vi "Get-velocity-profile.vi"(8 "error in (no error)":errorcluster, 11 "Motor-Maxon in":refnum<class "Motor-Maxon.lvclass">) -> (0 "error out":errorcluster, 1 "Velocity":i32, 2 "Velocity profile":T1, 3 "Motor-Maxon out":refnum<class "Motor-Maxon.lvclass">)   [LabVIEW 2013, in "PowderDeposition.lvlib" / "Motor-Maxon.lvclass"]
uses:
  Motor-Maxon.lvclass
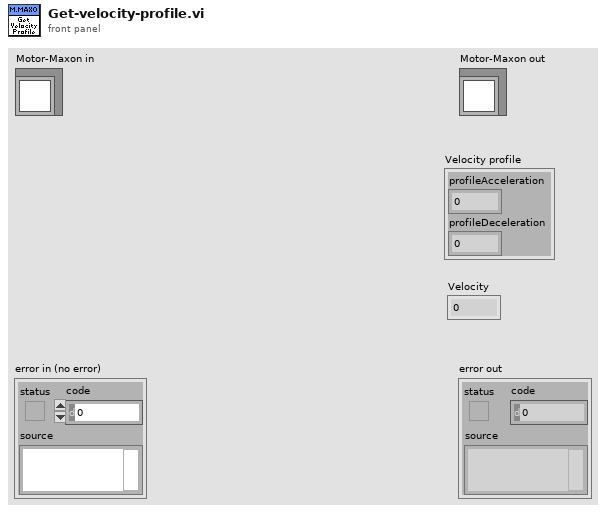
[diagram p1: front panel]
types:
  T1 = cluster{"profileAcceleration":u32, "profileDeceleration":u32}
  T2 = typedef "PowderDeposition.lvlib/Motor.lvclass/Action-settings.ctl" = cluster{"Speed":dbl, "Acceleration":dbl, "Direction":enum16{"Clockwise", "Counter-clockwise"}}
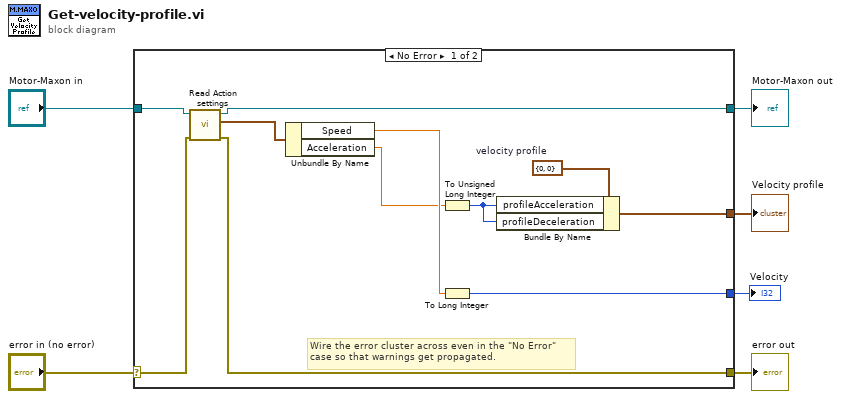
[diagram p0: block diagram]
diagram:
  n1 = case shown="No Error" "error in (no error)" {
    selector: "error in (no error)" -> [w10 w19]
    tunnel: [w9 w19] -> w5
    tunnel: [w16 w18] -> w3
    tunnel: "Motor-Maxon in" -> [w17 w18]
    tunnel: [w8 _] -> w1
    tunnel: [w7 _] -> w2
    frame No Error {
      w14 = T1 {"profileAcceleration"=0, "profileDeceleration"=0}  # velocity profile
      # "Wire the error cluster across even in the \"No Error\"\ncase so that warnings get propagated."
      n2 = call-dynamic "Read Action settings.vi"("error in (no error)"=w10, "Motor in"=w17) -> ("error out"=w9:errorcluster, "Action settings"=w15:T2, "Motor out"=w16:refnum<class "Motor-Maxon.lvclass">)  [unwired: 7 in]
      n3 = Unbundle By Name(w15) -> ("Speed"=w13:dbl, "Acceleration"=w12:dbl)
      n4 = To Unsigned Long Integer(number=w12) -> (unsigned 32bit integer=w11:u32)
      n5 = To Long Integer(number=w13) -> (32bit integer=w7:i32)
      n6 = Bundle By Name(cluster=w14, "profileAcceleration"=w11, "profileDeceleration"=w11) -> (w8:T1)
    }
    frame Error {
    }
  }
  "error out" <- w5
  "Motor-Maxon out" <- w3
  "Velocity profile" <- w1
  "Velocity" <- w2
